vi "analog_cache_with_timeout.vi"(3 "timeout":u32, 4 "valid":bool, 5 "analog_in":fxp<+/-,24,5>) -> (1 "timed_out":bool, 2 "$vall":fxp<+/-,24,5>)   [LabVIEW 2018]
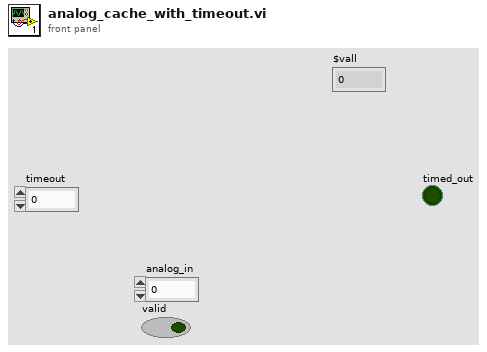
[diagram p1: front panel]
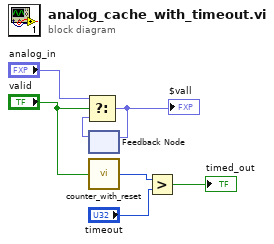
[diagram p0: block diagram]
diagram:
  n1 = feedback #1() -> (w6:fxp<+/-,24,5>)  [unwired: 1 in]
  n2 = Select(t="analog_in", s="valid", f=w6) -> (s? t:f=w7:fxp<+/-,24,5>)
  "$vall" <- w7
  n3 = feedback-in #1(w7) -> ()
  n4 = call "counter_with_reset.vi"("reset"="valid") -> ("count"=w3:u32)
  n5 = Greater?(x=w3, y="timeout") -> (0:→"timed_out":bool)
